vi "Priority.vi"(8 "error in (no error)":errorcluster, 11 "Caching in":refnum<class "Caching.lvclass">) -> (0 "error out":errorcluster, 2 "Priority":u16, 3 "Caching out":refnum<class "Caching.lvclass">)   [LabVIEW 2020, in "HTTP Server.lvlib" / "Caching.lvclass"]
uses:
  Caching.lvclass
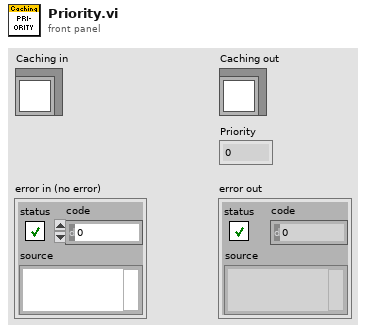
[diagram p1: front panel]
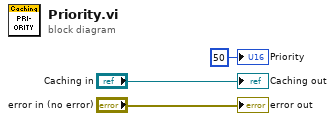
[diagram p0: block diagram]
diagram:
  "error out" <- "error in (no error)"
  "Caching out" <- "Caching in"
  "Priority" <- u16 50 ("Priority")
